vi "Make Window Always on Top.vi"(8 "error in (no error)":errorcluster, 9 "Activate? (F)":bool, 10 "window name (\"\")":string, 11 "window refnum":T1) -> (0 "error out":errorcluster, 3 "window refnum out":T1)   [LabVIEW 2020, in "MacroAssert.lvlib" / "Win Util.lvlib"]
doc: "This function will make the window named in the 'window name' input, or identified by the 'window refnum' the topmost window, so it will always be on top of other windows. If 'not a window refnum' is passed in, then the function will use the window name to get a window window refnum. If the window cannot be found, an error will be returned."
uses:
  Win Util.lvlib
  Window Refnum.ctl
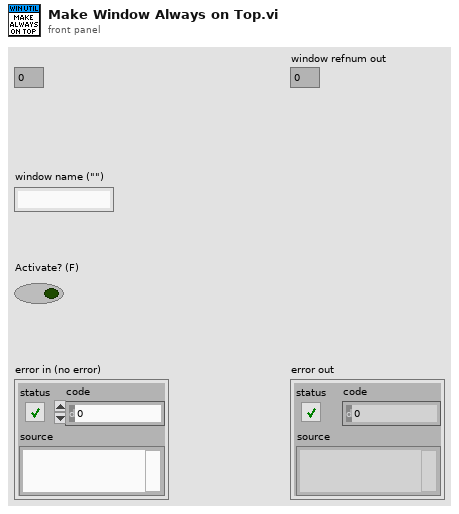
[diagram p1: front panel]
types:
  T1 = typedef "MacroAssert.lvlib/Win Util.lvlib/Window Refnum.ctl" = u64
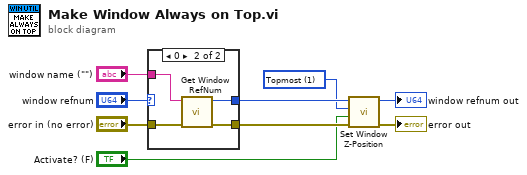
[diagram p0: block diagram]
diagram:
  w1 = u16 1 items=["Not Topmost", "Topmost", "Top", "Bottom"]
  n1 = case shown="0" "window refnum" {
    selector: "window refnum" -> [w10 _]
    tunnel: "error in (no error)" -> [w11 w15]
    tunnel: [w10 w14] -> w6
    tunnel: [w11 w13] -> w7
    tunnel: "window name (\"\")" -> [_ w12]
    frame Default {
    }
    frame 0 {
      n2 = call "Get Window RefNum.vi"("error in (no error)"=w15, "window name (\"\")"=w12) -> ("error out"=w13:errorcluster, "window refnum (NaWR)"=w14:T1)  [unwired: 6 out]
    }
  }
  n3 = call "Set Window Z-Position.vi"("error in (no error)"=w7, "No Activate? (F)"="Activate? (F)", "z-order position"=w1, "window refnum"=w6) -> ("error out"=→"error out":errorcluster, "window refnum out"=→"window refnum out":T1)  [unwired: 6 in]
